vi "PrepareAndSendSetROI.vi"(8 "error in (no error)":errorcluster, 9 "Clear ROI?(F)":bool=TRUE, 10 "ROI":T1, 11 "DisplayerUI in":refnum<class "DisplayerUI.lvclass">) -> (0 "error out":errorcluster, 3 "DisplayerUI out":refnum<class "DisplayerUI.lvclass">)   [LabVIEW 2020, in "DisplayerUI.lvlib" / "DisplayerUI.lvclass"]
uses:
  DisplayerUI.lvclass
  C:/Program Files/National Instruments/LabVIEW 2020/vi.lib/ActorFramework/Actor/Actor.lvclass
  Hardware Abstraction Layer/Component/Device/Device/DataExchange.ctl
  <vilib>/ActorFramework/Actor/Actor.lvclass/Actor.ctl
  DisplayerUI.lvclass/DisplayerUI.ctl
  Interface/DataListener Messages/OnDataChange Msg/OnDataChange Msg.lvclass/OnDataChange Msg.ctl
  <vilib>/ActorFramework/Message Enqueuer/Message Enqueuer.lvclass/Message Enqueuer.ctl
  <vilib>/ActorFramework/Message Enqueuer/Enqueue.vi
  Interface/DataListener Messages/OnDataChange Msg/OnDataChange Msg.lvclass
  C:/Program Files/National Instruments/LabVIEW 2020/vi.lib/ActorFramework/Message/Message.lvclass
  <vilib>/ActorFramework/Message Priority Queue/Priority Enqueue.vi
  <vilib>/ActorFramework/Actor/Actor.lvclass
  Interface/DataListener/DataListener.lvclass
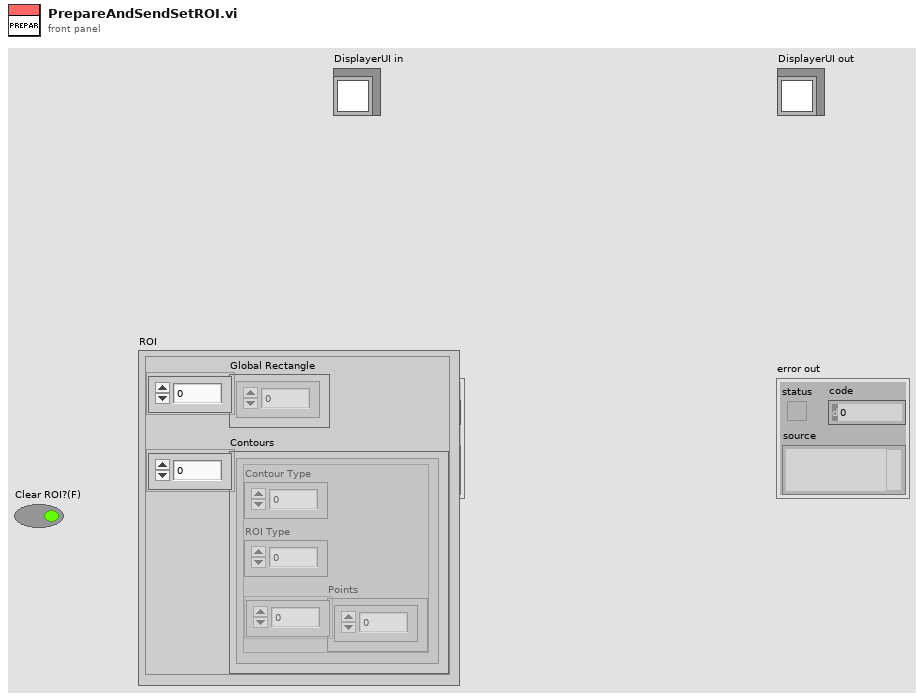
[diagram p1: front panel]
types:
  T1 = cluster{"Global Rectangle":i32[], "Contours":cluster{"Contour Type":u32, "ROI Type":u32, "Points":i32[]}[]}
  T2 = typedef "DataListener.lvclass/DataExchange.ctl" = cluster{"Source":string, "Destination":string, "Description":string, "value":variant}
  T3 = cluster{"x":dbl, "y":dbl, "width":dbl, "height":dbl}
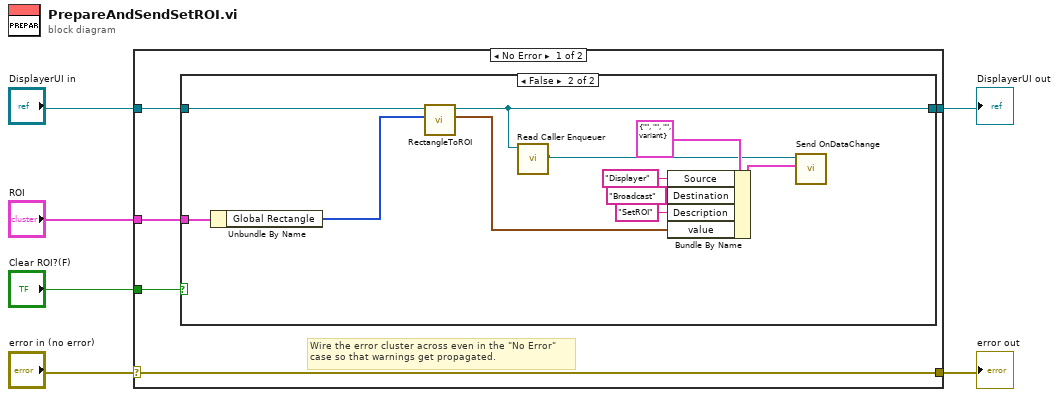
[diagram p0: block diagram]
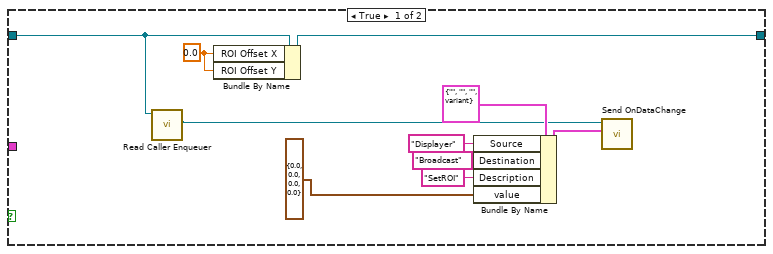
[diagram p2: hidden frame]
diagram:
  n1 = case shown="No Error" "error in (no error)" {
    selector: "error in (no error)" -> [w11 w34]
    tunnel: [w11 w34] -> w1
    tunnel: [w8 w33] -> w2
    tunnel: "DisplayerUI in" -> [w9 w33]
    tunnel: "ROI" -> [w10 _]
    tunnel: "Clear ROI?(F)" -> [w7 _]
    frame No Error {
      # "Wire the error cluster across even in the \"No Error\"\ncase so that warnings get propagated."
      n2 = case shown="False" w7 {
        tunnel: w10 -> [_ w32]
        tunnel: w9 -> [w19 w31]
        tunnel: [w21 w29] -> w8
        frame True {
          w20 = 0.0 ("ROI Offset X")
          n3 = call <vilib>:"Read Caller Enqueuer.vi"("Actor"=w19) -> ("Caller Enqueuer"=w13:refnum<class "Message Enqueuer.lvclass">)  [unwired: 10 in]
          n4 = Bundle By Name(cluster=w19, "ROI Offset X"=w20, "ROI Offset Y"=w20) -> (w21:refnum<class "DisplayerUI.lvclass">)
          n5 = Bundle By Name(cluster=T2 {"Source"="", "Destination"="", "Description"="", "value"=variant} ("DataExchange"), "Source"="Displayer", "Destination"="Broadcast", "Description"="SetROI", "value"=T3 {"x"=0.0, "y"=0.0, "width"=0.0, "height"=0.0} ("Setting.ROI")) -> (w17:T2)
          n6 = call "Send OnDataChange.vi"("DataExchange"=w17, "Message Enqueuer"=w13) -> ()  [unwired: 8 in, 2 out]
        }
        frame False {
          n7 = Unbundle By Name(w32) -> ("Global Rectangle"=w30:i32[])
          n8 = call-dynamic "RectangleToROI.vi"("Global Rectangle in"=w30, "DisplayerUI in"=w31) -> ("Setting.ROI"=w22:T3, "DisplayerUI out"=w29:refnum<class "DisplayerUI.lvclass">)  [unwired: 7 in, 1 out]
          n9 = call <vilib>:"Read Caller Enqueuer.vi"("Actor"=w29) -> ("Caller Enqueuer"=w23:refnum<class "Message Enqueuer.lvclass">)  [unwired: 10 in]
          n10 = Bundle By Name(cluster=T2 {"Source"="", "Destination"="", "Description"="", "value"=variant} ("DataExchange"), "Source"="Displayer", "Destination"="Broadcast", "Description"="SetROI", "value"=w22) -> (w27:T2)
          n11 = call "Send OnDataChange.vi"("DataExchange"=w27, "Message Enqueuer"=w23) -> ()  [unwired: 8 in, 2 out]
        }
      }
    }
    frame Error {
    }
  }
  "error out" <- w1
  "DisplayerUI out" <- w2
